vi "Enqueue Message (Array) - Q1 Create SV.vi"(8 "error in (no error)":errorcluster, 10 "Message Array":T1[](array[typedef]), 11 "Qin":refnum<queue>) -> (0 "error out":errorcluster, 3 "Qout":refnum<queue>)   [LabVIEW 2014]
doc: "For a regular message, enqueue the message. For a priority message, enqueue it at the front of the queue."
uses:
  TypeDef/Q1 Create SV.ctl
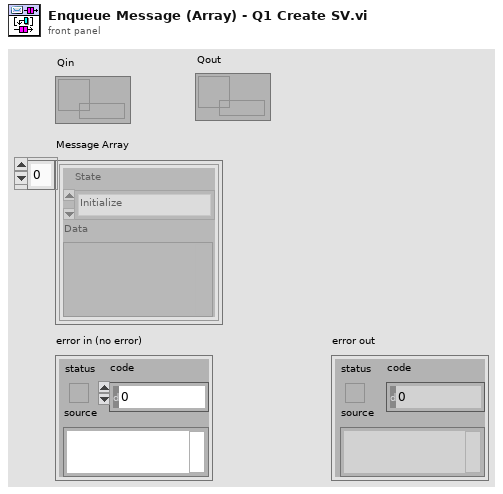
[diagram p1: front panel]
types:
  T1 = typedef "Q1 Create SV.ctl" = cluster{"State":enum16{"Initialize", "Idle", "Prepare", "Create", "Save Library", "Bind SV", "Exit", "Error", "Save Project", "Check Library Name"}, "Data":variant}
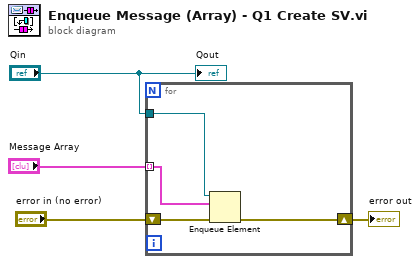
[diagram p0: block diagram]
diagram:
  n1 = for {
    tunnel: "Qin" -> [w6]
    shift-right: [w7] -> w3
    shift-left: "error in (no error)" -> [w8]
    tunnel: "Message Array" -> [w5] mode=indexing
    n2 = Enqueue Element(queue=w6, element=w5, error in (no error)=w8) -> (error out=w7:errorcluster)  [unwired: 1 in, 2 out]
  }
  "error out" <- w3
  "Qout" <- "Qin"
